vi "Base 10 Digit Count.vi"(11 "number":i32) -> (3 "digit count":i32)   [LabVIEW 2017, in "DSF Core.lvlib"]
uses:
  DSF Core.lvlib
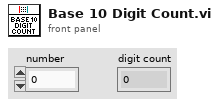
[diagram p1: front panel]
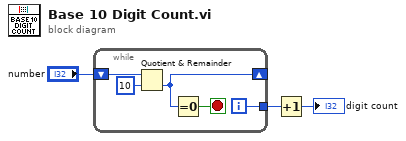
[diagram p0: block diagram]
diagram:
  n1 = while {
    shift-right: [w6] -> _
    shift-left: "number" -> [w8]
    tunnel: [w4] -> w2
    i -> [w4]
    stop <- w5 stop-if-true
    n2 = Quotient & Remainder(x=w8, y=10) -> (floor(x/y)=w6:i32)  [unwired: 1 out]
    n3 = Equal To 0?(x=w6) -> (x = 0?=w5:bool)
  }
  n4 = Increment(x=w2) -> (x+1=→"digit count":i32)
